vi "Select_devices.vi"(8 "error in (no error)":errorcluster {"code" format="%.0x"}, 10 "Number of devices":u32) -> (0 "error out":errorcluster {"code" format="%.0x"}, 3 "PM ResourceName Out":string)   [LabVIEW 2021]
doc: "This VI enables to get the list of the USB devices.\n\nInputs:\n(1) Number of devices - the number of devices (according to the TLPM library).\n(2) Error in.\n\nOutputs:\n(1) PM ResourceName Out - the list of the devices.\n(2) Error out."
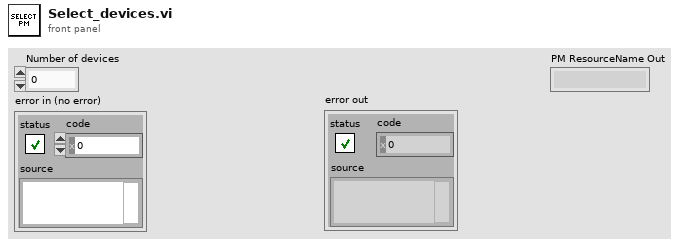
[diagram p1: front panel]
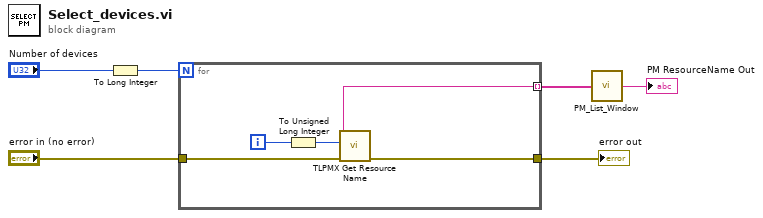
[diagram p0: block diagram]
diagram:
  n1 = To Long Integer(number="Number of devices") -> (32bit integer=w2:i32)
  n2 = for {
    N: w2 -> [_]
    tunnel: "error in (no error)" -> [w8]
    tunnel: [w10] -> w5
    tunnel: [w9] -> w4 mode=indexing
    i -> [w11]
    n3 = To Unsigned Long Integer(number=w11) -> (unsigned 32bit integer=w7:u32)
    n4 = call "TLPMX Get Resource Name.vi"("error in (no error)"=w8, "Index (0)"=w7) -> ("error out"=w10:errorcluster, "Resource Name"=w9:string)  [unwired: 7 in, 1 out]
  }
  "error out" <- w5
  n5 = call "PM_List_Window.vi"("Array"=w4) -> ("Resource Name Out"=→"PM ResourceName Out":string)  [unwired: 4 in]
